vi "Set Manifold Channel.vi"(8 "error in":errorcluster, 9 "On/Off":bool, 10 "Manifold Channel":i32, 11 "Gantry in":refnum<class "Gantry.lvclass">) -> (0 "error out":errorcluster, 3 "Gantry out":refnum<class "Gantry.lvclass">)   [LabVIEW 2017, in "Gantry.lvclass"]
uses:
  Gantry.lvclass
  <vilib>/DAQmx/write.llb/DAQmx Write (Digital 1D Bool 1Chan 1Samp).vi
  <vilib>/DAQmx/miscellaneous.llb/DAQmx Fill In Error Info.vi
  FlexWorktable/FlexWorktable.lvclass
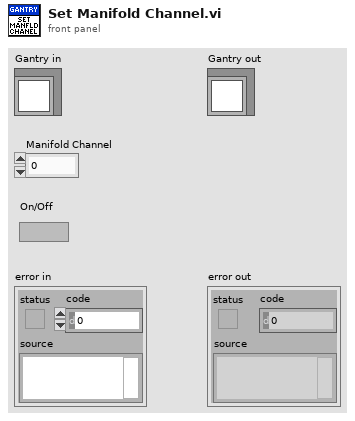
[diagram p1: front panel]
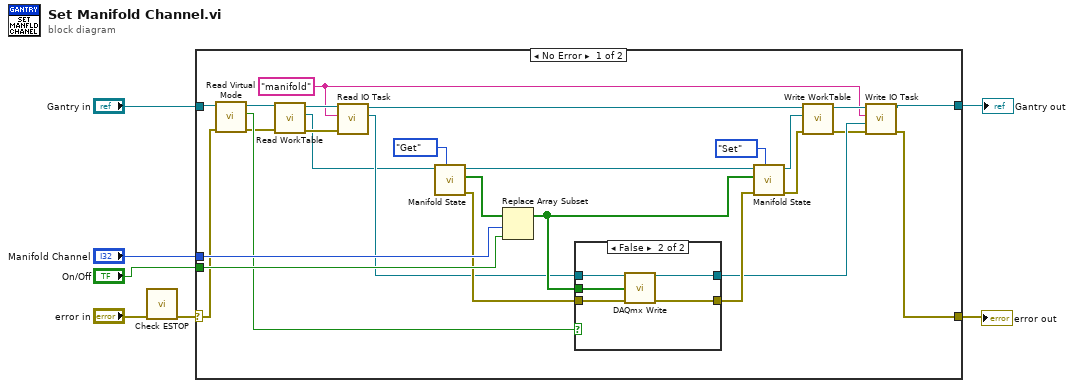
[diagram p0: block diagram]
diagram:
  n1 = call "Check ESTOP.vi"("error in"="error in") -> ("error out"=w2:errorcluster)  [unwired: 10 in]
  n2 = case shown="No Error" w2 {
    selector: w2 -> [w21 w43]
    tunnel: [w8 w43] -> w7
    tunnel: [w9 w42] -> w6
    tunnel: "Gantry in" -> [w32 w42]
    tunnel: "Manifold Channel" -> [w34 _]
    tunnel: "On/Off" -> [w33 _]
    frame No Error {
      w14 = "manifold" ("Task Name")
      n3 = call-dynamic "Read Virtual Mode.vi"("error in (no error)"=w21, "Gantry in"=w32) -> ("error out"=w20:errorcluster, "Is Virtual"=w31:bool, "Gantry out"=w23:refnum<class "Gantry.lvclass">)  [unwired: 6 in, 1 out]
      n4 = call-dynamic "Read WorkTable.vi"("error in"=w20, "Gantry Class in"=w23) -> ("error out"=w19:errorcluster, "Worktable"=w17:refnum<class "FlexWorktable.lvclass">, "Gantry Class out"=w22:refnum<class "Gantry.lvclass">)  [unwired: 7 in]
      n5 = call "Read IO Task.vi"("error in (no error)"=w19, "Task Name"=w14, "Gantry in"=w22) -> ("task/channels in"=w18:refnum<k21>, "Gantry out"=w16:refnum<class "Gantry.lvclass">)  [unwired: 6 in, 1 out]
      n6 = call-dynamic "Manifold State.vi"("Get/Set"=enum16{"Get", "Set"}."Get", "FlexWorktable in"=w17) -> ("error out"=w29:errorcluster, "State"=w26:bool[], "FlexWorktable out"=w28:refnum<class "FlexWorktable.lvclass">)  [unwired: 7 in]
      n7 = Replace Array Subset(array=w26, new element=w33, index=w34) -> (w25:bool[])
      n8 = case shown="False" w31 {
        tunnel: [w36 w41] -> w24
        tunnel: w25 -> [_ w40]
        tunnel: w18 -> [w35 w39]
        tunnel: w29 -> [w36 w38]
        tunnel: [w35 w37] -> w13
        frame True {
        }
        frame False {
          n9 = call-poly <vilib>:"DAQmx Write.vi"("task/channels in"=w39, "data"=w40, "error in"=w38) -> ("task out"=w37:refnum<k21>, "error out"=w41:errorcluster)  [unwired: 10 in, 1 out]
        }
      }
      n10 = call-dynamic "Manifold State.vi"("Get/Set"=enum16{"Get", "Set"}."Set", "error in (no error)"=w24, "New State"=w25, "FlexWorktable in"=w28) -> ("error out"=w11:errorcluster, "FlexWorktable out"=w12:refnum<class "FlexWorktable.lvclass">)  [unwired: 5 in, 1 out]
      n11 = call-dynamic "Write WorkTable.vi"("error in (no error)"=w11, "FlexWorktable"=w12, "Gantry Class in"=w16) -> ("error out"=w10:errorcluster, "Gantry Class out"=w15:refnum<class "Gantry.lvclass">)  [unwired: 7 in]
      n12 = call "Write IO Task.vi"("error in (no error)"=w10, "IO Task"=w13, "Task Name"=w14, "Gantry in"=w15) -> ("error out"=w8:errorcluster, "Gantry out"=w9:refnum<class "Gantry.lvclass">)  [unwired: 6 in]
    }
    frame Error {
    }
  }
  "error out" <- w7
  "Gantry out" <- w6
